vi "Ballard XML Generator.Open Core.vi"(9 "name":string, 10 "id":i32, 11 "string in":string) -> (3 "string out":string)   [LabVIEW 2017]
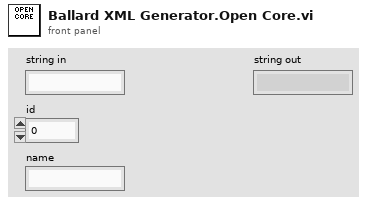
[diagram p1: front panel]
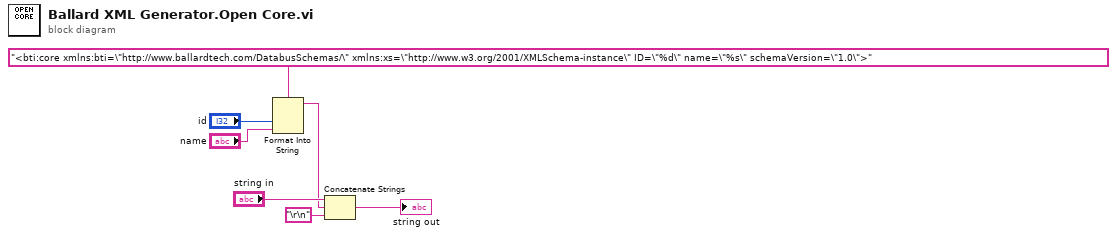
[diagram p0: block diagram]
diagram:
  n1 = Format Into String(format string="<bti:core xmlns:bti=\"http://www.ballardtech.com/DatabusSchemas/\" xmlns:xs=\"http://www.w3.org/2001/XMLSchema-instance\" ID=\"%d\" name=\"%s\" schemaVersion=\"1.0\">", "id", "name") -> (resulting string=w1:string)  [unwired: 2 in, 1 out]
  n2 = Concatenate Strings("string in", w1, "\r\n") -> (→"string out":string)
